vi "Write I32.vi"(8 "error in":errorcluster, 9 "value in":i32, 10 "register offset":u32, 11 "session in":u32) -> (0 "error out":errorcluster, 3 "session out":u32)   [LabVIEW 2018, in "Scalar IO Operations.lvlib"]
uses:
  Scalar IO Operations.lvlib
  NiFpga.dll
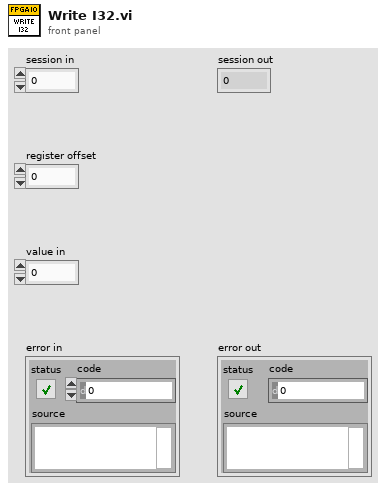
[diagram p1: front panel]
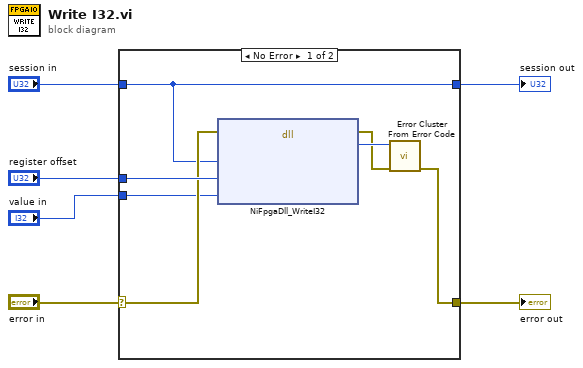
[diagram p0: block diagram]
diagram:
  n1 = case shown="No Error" "error in" {
    selector: "error in" -> [w12 w15]
    tunnel: "session in" -> [w11 w14]
    tunnel: [w7 w15] -> w5
    tunnel: "register offset" -> [w13 _]
    tunnel: [w11 w14] -> w2
    tunnel: "value in" -> [w10 _]
    frame No Error {
      n2 = dll-call lib="NiFpga.*" fn="NiFpgaDll_WriteI32"(error in=w12, "session"=w11, "offset"=w13, "value"=w10) -> (error out=w8:errorcluster, "status"=w9:i32)  [unwired: 5 in, 1 out]
      n3 = call <vilib>:"Error Cluster From Error Code.vi"("error in (no error)"=w8, "error code (0)"=w9) -> ("error out"=w7:errorcluster)  [unwired: 7 in]
    }
    frame Error {
    }
  }
  "error out" <- w5
  "session out" <- w2
